vi "Set Test Step .vi"(8 "error in (no error)":errorcluster, 10 "Sequence Context In":refnum<k7>, 11 "TestExec.lvclass":refnum<class "TestExec.lvclass">) -> (0 "error out":errorcluster, 1 "Test Running":bool, 2 "Next Step":i32, 3 "TestExec.lvclass":refnum<class "TestExec.lvclass">, 4 "HV":bool)   [LabVIEW 2019, in "OPC UA.lvlib" / "TestExec.lvclass"]
uses:
  TestExec.lvclass
  C:/Workspace/BSM OOP/Sequence/CodeModules/OPC UA Client/OPC UA/OPC UA.lvclass
  OPC UA/OPC UA.lvclass/OPC UA.ctl
  <vilib>/addons/TestStand/_TSUtility.llb/TestStand - Set Property Value (Number {Unsigned 32-bit Integer}).vi
  OPC UA/OPC UA.lvclass
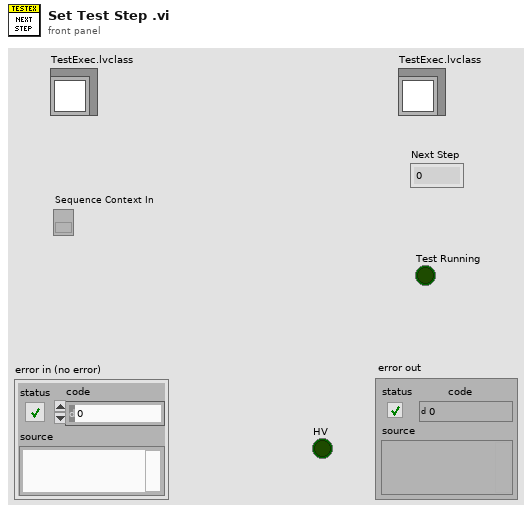
[diagram p1: front panel]
types:
  T1 = typedef "OPC UA.lvlib/OPC UA.lvclass/Tester Rx Dataset.ctl" = cluster{"Start":bool, "NestStatus":bool, "PalletID":u32, "BarcodeData":string, "StepEcho":u32, "Cylinder_1":bool, "Cylinder_2":bool, "Cylinder_3":bool, "Cylinder_4":bool, "Cylinder_5":bool, "ResultsAck":bool, "Reset":bool, "Stop":bool, "FaultCode":u32}
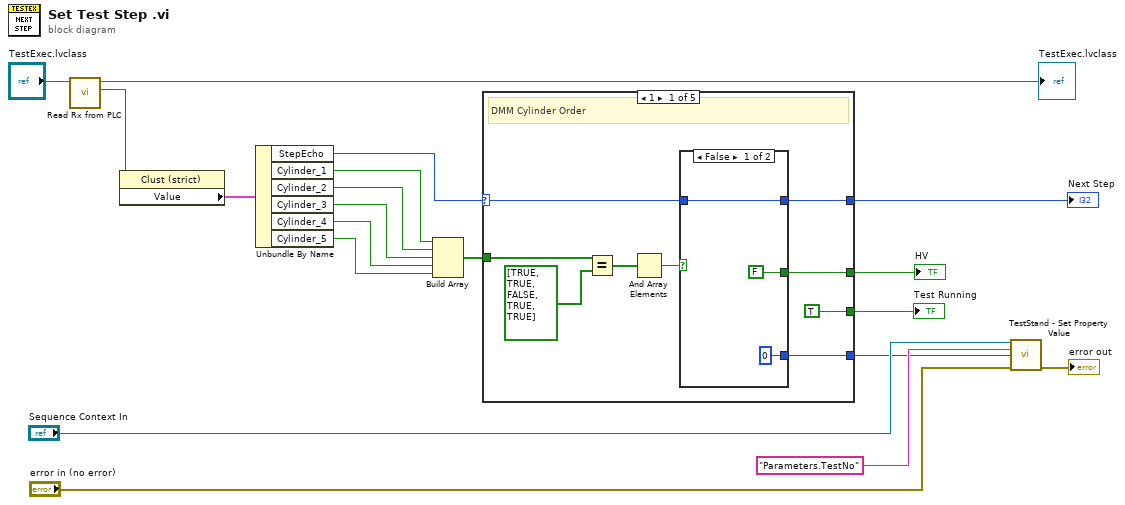
[diagram p0: block diagram]
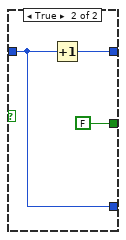
[diagram p2: hidden frame]
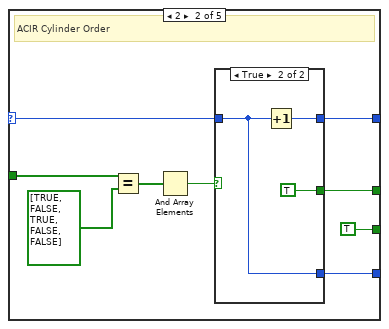
[diagram p3: hidden frame]
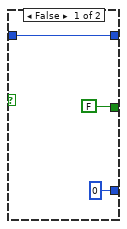
[diagram p4: hidden frame]
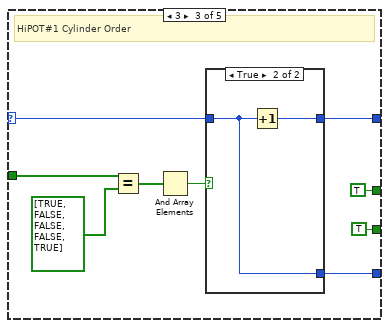
[diagram p5: hidden frame]
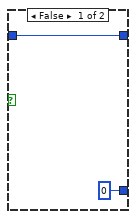
[diagram p6: hidden frame]
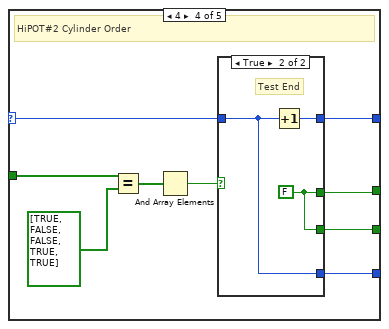
[diagram p7: hidden frame]
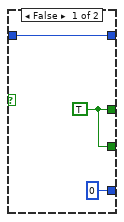
[diagram p8: hidden frame]
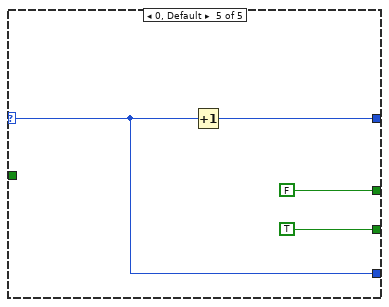
[diagram p9: hidden frame]
diagram:
  n1 = call "Read Rx from PLC.vi"("OPC UA in"="TestExec.lvclass") -> ("Rx from PLC"=w8:refnum<vi>, "OPC UA out"=→"TestExec.lvclass":refnum<class "TestExec.lvclass">)  [unwired: 8 in, 1 out]
  n2 = property class="Clust (strict)"(reference=w8) -> ("Value"=w7:T1)  [unwired: 1 in, 2 out]
  n3 = Unbundle By Name(w7) -> ("StepEcho"=w6:u32, "Cylinder_1"=w5:bool, "Cylinder_2"=w4:bool, "Cylinder_3"=w3:bool, "Cylinder_4"=w2:bool, "Cylinder_5"=w1:bool)
  n4 = Build Array(w5, w4, w3, w2, w1) -> (w19:bool[])
  n5 = case shown="1" w6 {
    selector: w6 -> [w26 w40 w54 w64 w78]
    tunnel: w19 -> [w21 w36 w51 w70 _]
    tunnel: [w23 w39 w53 w63 w79] -> w18
    tunnel: [w24 w38 TRUE w67 FALSE] -> w17
    tunnel: [TRUE ("Test Running") TRUE ("Test Running") TRUE ("Test Running") w66 TRUE ("Test Running")] -> w16
    tunnel: [w20 w35 w52 w65 w78] -> w11
    frame 1 {
      # "DMM Cylinder Order"
      n6 = Equal?(x=w21, y=bool[] [TRUE, TRUE, FALSE, TRUE, TRUE]) -> (x = y?=w28:bool[])
      n7 = And Array Elements(Boolean array=w28) -> (logical AND=w25:bool)
      n8 = case shown="False" w25 {
        tunnel: w26 -> [w30 w32]
        tunnel: [w30 w34] -> w23
        tunnel: [FALSE FALSE] -> w24
        tunnel: [u32 0 ("StepEcho") w32] -> w20
        frame False {
        }
        frame True {
          n9 = Increment(x=w32) -> (x+1=w34:u32)
        }
      }
    }
    frame 2 {
      # "ACIR Cylinder Order"
      n10 = Equal?(x=w36, y=bool[] [TRUE, FALSE, TRUE, FALSE, FALSE]) -> (x = y?=w43:bool[])
      n11 = And Array Elements(Boolean array=w43) -> (logical AND=w41:bool)
      n12 = case shown="True" w41 {
        tunnel: w40 -> [w45 w47]
        tunnel: [w45 w49] -> w39
        tunnel: [FALSE TRUE] -> w38
        tunnel: [u32 0 ("StepEcho") w47] -> w35
        frame False {
        }
        frame True {
          n13 = Increment(x=w47) -> (x+1=w49:u32)
        }
      }
    }
    frame 3 {
      # "HiPOT#1 Cylinder Order"
      n14 = Equal?(x=w51, y=bool[] [TRUE, FALSE, FALSE, FALSE, TRUE]) -> (x = y?=w58:bool[])
      n15 = And Array Elements(Boolean array=w58) -> (logical AND=w55:bool)
      n16 = case shown="True" w55 {
        tunnel: w54 -> [w60 w61]
        tunnel: [w60 w62] -> w53
        tunnel: [u32 0 ("StepEcho") w61] -> w52
        frame False {
        }
        frame True {
          n17 = Increment(x=w61) -> (x+1=w62:u32)
        }
      }
    }
    frame 4 {
      # "HiPOT#2 Cylinder Order"
      n18 = Equal?(x=w70, y=bool[] [TRUE, FALSE, FALSE, TRUE, TRUE]) -> (x = y?=w71:bool[])
      n19 = And Array Elements(Boolean array=w71) -> (logical AND=w68:bool)
      n20 = case shown="True" w68 {
        tunnel: [w74 w77] -> w67
        tunnel: [w74 w77] -> w66
        tunnel: [u32 0 ("StepEcho") w76] -> w65
        tunnel: w64 -> [w73 w76]
        tunnel: [w73 w75] -> w63
        frame False {
          w74 = TRUE
        }
        frame True {
          w77 = FALSE
          # "Test End"
          n21 = Increment(x=w76) -> (x+1=w75:u32)
        }
      }
    }
    frame 0, Default {
      n22 = Increment(x=w78) -> (x+1=w79:u32)
    }
  }
  "Next Step" <- w18
  "HV" <- w17
  "Test Running" <- w16
  n23 = call-poly <vilib>:"TestStand - Set Property Value.vi"("Sequence Context In"="Sequence Context In", "Lookup String"="Parameters.TestNo", "New Value"=w11, "error in (no error)"="error in (no error)") -> ("error out"=→"error out":errorcluster)  [unwired: 10 in, 1 out]
